vi "Save2009.vi"   [LabVIEW 2013]
uses:
  <vilib>/Heliosphere Research LLC/Advanced Plotting Toolkit/Advanced Plotting Toolkit.lvlib
types:
  T1 = typedef "Advanced Plotting Toolkit.lvlib/PlotID.ctl" = i32
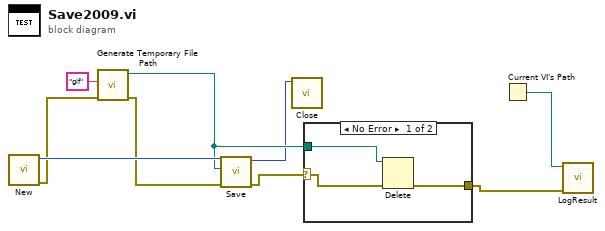
[diagram p0: block diagram]
diagram:
  n1 = call <vilib>:"New.vi"() -> ("error out"=w6:errorcluster, "Plot ID"=w7:T1)  [unwired: 10 in]
  n2 = call <vilib>:"Generate Temporary File Path.vi"("error in (no error)"=w6, "Temporary File Extension (tmp)"="gif") -> ("error out"=w5:errorcluster, "Unique Temporary File Path"=w3:path)  [unwired: 8 in]
  n3 = call <vilib>:"Save.vi"("error in (no error)"=w5, "Path"=w3, "Plot ID In"=w7) -> ("error out"=w4:errorcluster, "Plot ID Out"=w1:T1)  [unwired: 7 in]
  n4 = call <vilib>:"Close.vi"("Plot ID"=w1) -> ()  [unwired: 11 in]
  n5 = case shown="No Error" w4 {
    selector: w4 -> [w11 w13]
    tunnel: w3 -> [w12 _]
    tunnel: [w10 w13] -> w2
    frame No Error {
      n6 = Delete(path (use dialog)=w12, error in=w11) -> (error out=w10:errorcluster)  [unwired: 3 in, 2 out]
    }
    frame Error {
    }
  }
  n7 = Current VI's Path() -> (path=w9:path)
  n8 = call "LogResult.vi"("Test Result"=w2, "VI Path"=w9) -> ()  [unwired: 10 in]
